vi "Set Data Version.vi"(8 "error in (no error)":errorcluster, 10 "data version":T1, 11 "Configuration in":refnum<class "Configuration.lvclass">) -> (0 "error out":errorcluster, 3 "Configuration out":refnum<class "Configuration.lvclass">)   [LabVIEW 2017]
uses:
  Configuration.lvclass
  Typedefs/DSF Version Info.ctl
  DSF Core.lvlib
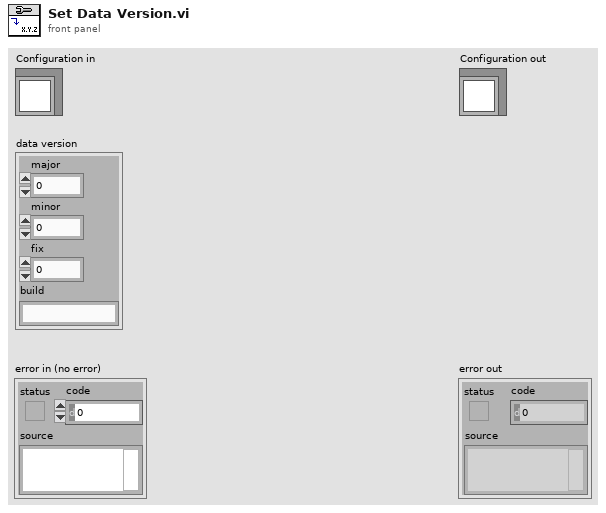
[diagram p1: front panel]
types:
  T1 = typedef "DSF Core.lvlib/DSF Version Info.ctl" = cluster{"major":i32, "minor":i32, "fix":i32, "build":string}
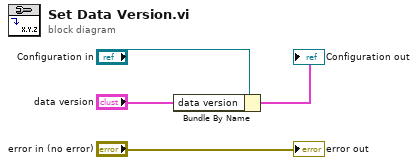
[diagram p0: block diagram]
diagram:
  n1 = Bundle By Name(cluster="Configuration in", "data version"="data version") -> (→"Configuration out":cluster{})
  "error out" <- "error in (no error)"
